vi "outline_boundaries_for_c_parameter.vi"(8 "Error In":errorcluster, 9 "Xi":T4, 10 "Sample":string, 11 "File Path":path) -> (0 "Error Out":errorcluster, 2 "Image":string, 3 "ROI":T1)   [LabVIEW 2019]
uses:
  xi_angles_enum_typedef.ctl
  image_property_cluster_typedef.ctl
  outline_boundaries_for_c_parameter_states_enum_typedef.ctl
  <vilib>/vision/NI_Vision_Development_Module.lvlib
panel:
  in  "Operator Value":sgl format="%.2f"
  in  "Operator":T2(ring)
  out "Image Properties":T3
  in  "Done":bool
  in  "Frame":i32(slide) min=0 max=19 step=1 scale=0.0..19.0
  out "Image":T5(plugin-control)
  # "Outline Boundaries for c-Parameter Determination"
  # "Use the open boundary selection tool to ouline grain boundaries that you wish to use for determining the c-parameter.\nRemember grains further from the center work the best for this task as they are more sensitive to the c-parameter."
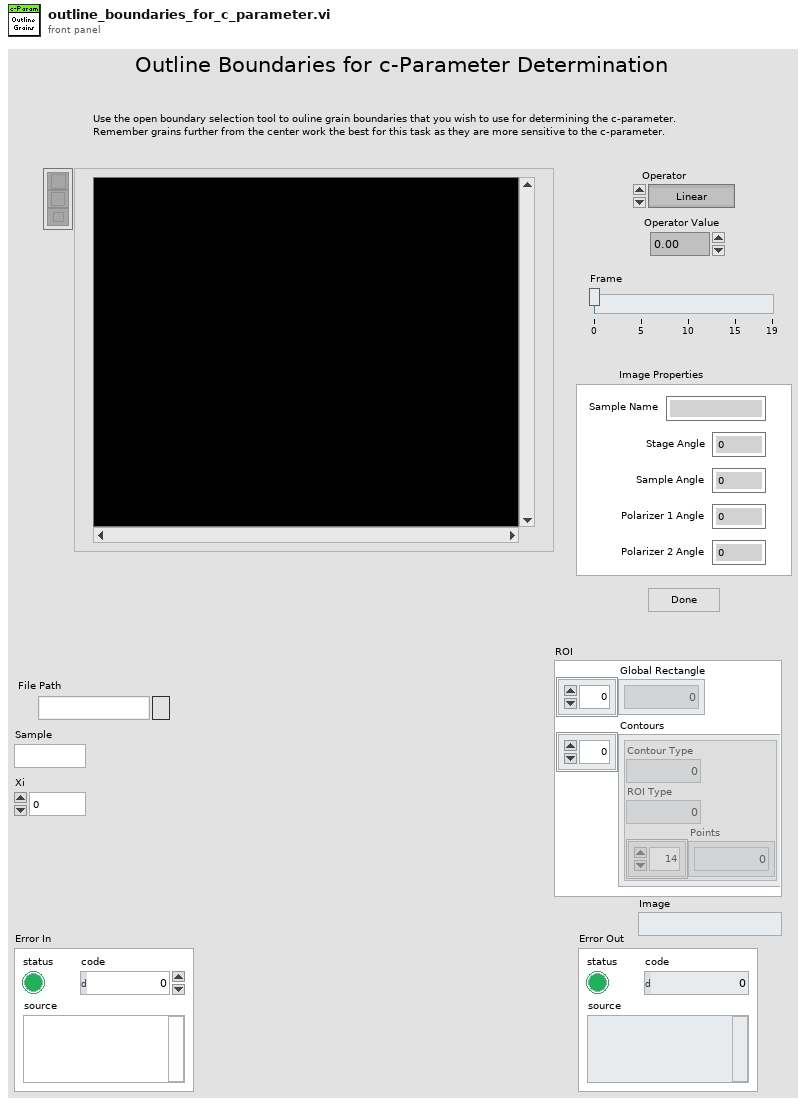
[diagram p1: front panel]
types:
  T1 = cluster{"Global Rectangle":i32[], "Contours":cluster{"Contour Type":u32, "ROI Type":u32, "Points":i32[]}[]}
  T2 = enum32{"Linear", "Log", "Exp", "Square", "Square root", "Power X", "Power 1/X"}
  T3 = typedef "image_property_cluster_typedef.ctl" = cluster{"Stage Angle":dbl, "Sample Angle":dbl, "Polarizer 1 Angle":dbl, "Polarizer 2 Angle":dbl, "Sample Name":string}
  T4 = typedef "xi_angles_enum_typedef.ctl" = enum16{"0", "45"}
  T5 = typedef "IMAQ Image.ctl" = refnum<image>
  T6 = typedef "outline_boundaries_for_c_parameter_states_enum_typedef.ctl" = enum16{"Enhance", "Plot Image", "Shutdown", "Wait", "Initialize", ""}
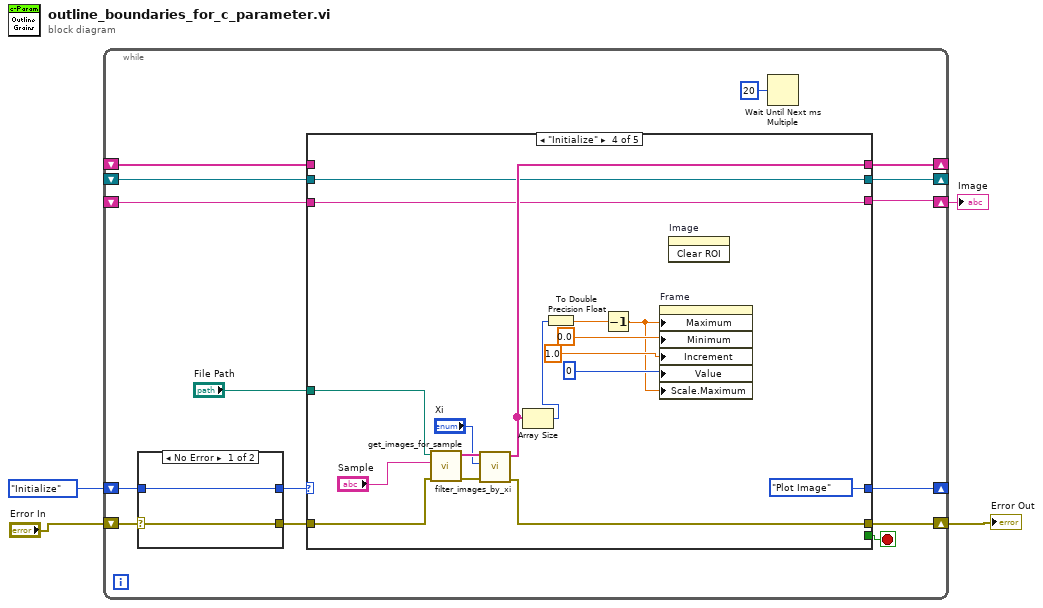
[diagram p0: block diagram]
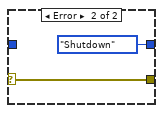
[diagram p2: hidden frame]
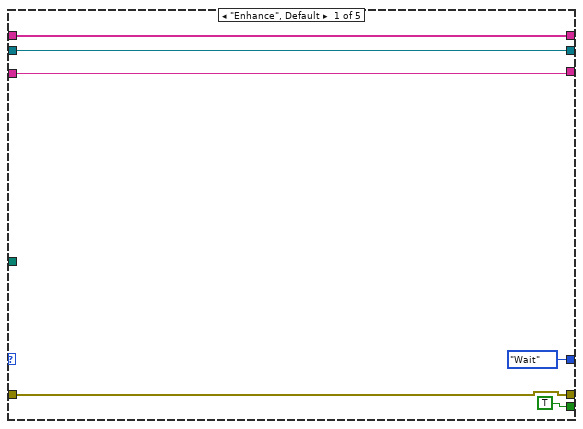
[diagram p3: hidden frame]
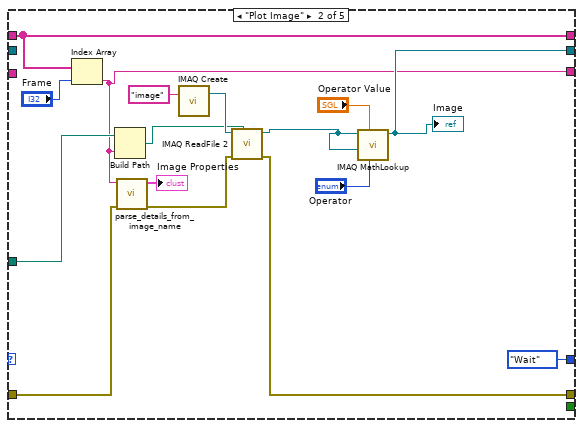
[diagram p4: hidden frame]
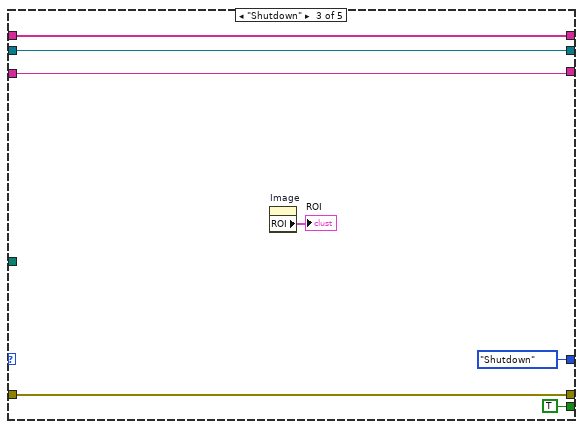
[diagram p5: hidden frame]
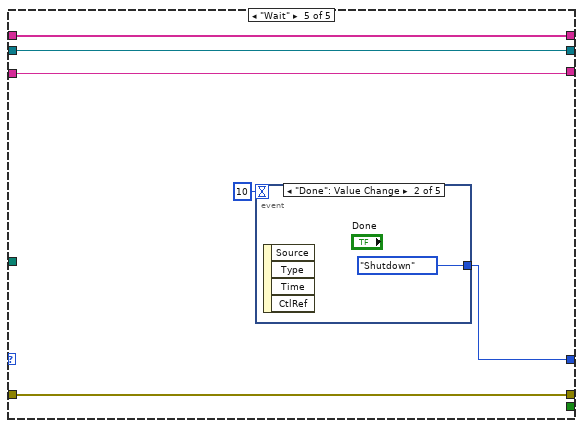
[diagram p6: hidden frame]
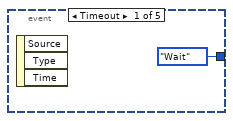
[diagram p7: hidden frame]
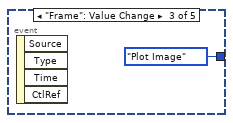
[diagram p8: hidden frame]
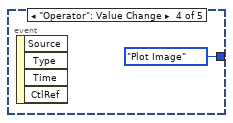
[diagram p9: hidden frame]
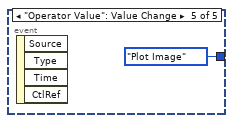
[diagram p10: hidden frame]
diagram:
  n1 = while {
    shift-right: [w16] -> _
    shift-left: outline_boundaries_for_c_parameter_states_enum_typedef."Initialize" -> [w19]
    shift-right: [w15] -> w2
    shift-left: "Error In" -> [w18]
    shift-right: [w13] -> _
    shift-left: _ -> [w12]
    shift-right: [w8] -> _
    shift-left: _ -> [w10]
    shift-right: [w6] -> w1
    shift-left: _ -> [w5]
    stop <- w14 stop-if-true
    n2 = case shown="No Error" w18 {
      selector: w18 -> [w20 w22]
      tunnel: [w21 outline_boundaries_for_c_parameter_states_enum_typedef."Shutdown"] -> w7
      tunnel: w19 -> [w21 _]
      tunnel: [w20 w22] -> w17
      frame No Error {
      }
      frame Error {
      }
    }
    n3 = case shown="\"Initialize\"" w7 {
      tunnel: w17 -> [w25 w35 w50 w65 w73]
      tunnel: [outline_boundaries_for_c_parameter_states_enum_typedef."Wait" outline_boundaries_for_c_parameter_states_enum_typedef."Wait" outline_boundaries_for_c_parameter_states_enum_typedef."Shutdown" outline_boundaries_for_c_parameter_states_enum_typedef."Plot Image" w74] -> w16
      tunnel: [w25 w40 w50 w59 w73] -> w15
      tunnel: [TRUE _ TRUE _ _] -> w14
      tunnel: [w27 w38 w52 w58 w72] -> w13
      tunnel: w12 -> [w27 w38 w52 _ w72]
      tunnel: "File Path" -> [_ w44 _ w57 _]
      tunnel: [w26 w31 w51 w56 w71] -> w8
      tunnel: w10 -> [w26 _ w51 w56 w71]
      tunnel: [w24 w30 w46 w53 w70] -> w6
      tunnel: w5 -> [w24 _ w46 w53 w70]
      frame "Enhance", Default {
      }
      frame "Plot Image" {
        n4 = Index Array(array=w38, index="Frame") -> (element=w30:string)
        n5 = Build Path(base path=w44, name or relative path=w30) -> (appended path=w41:path)
        n6 = call "parse_details_from_image_name.vi"("Error In"=w35, "Image Name"=w30) -> ("Error Out"=w36:errorcluster, "Image Properties"=→"Image Properties":T3)  [unwired: 8 in]
        n7 = call "IMAQ Create"("Image Name"="image") -> ("New Image"=w42:T5)  [unwired: 4 in, 1 out]
        n8 = call "IMAQ ReadFile 2"("File Path"=w41, "error in (no error)"=w36, "Image"=w42) -> ("error out"=w40:errorcluster, "Image Out"=w32:T5)  [unwired: 4 in, 3 out]
        n9 = call "IMAQ MathLookup"("Operator"="Operator", "X Value"="Operator Value", "Image Dst"=w32, "Image Src"=w32) -> ("Image Dst Out"=w31:T5)  [unwired: 6 in, 1 out]
        "Image" <- w31
      }
      frame "Shutdown" {
        n10 = property on="Image" class="ImageControl"() -> ("ROI"=→"ROI":T1)  [unwired: 2 in, 2 out]
      }
      frame "Initialize" {
        n11 = call "get_images_for_sample.vi"("Error In"=w65, "Sample"="Sample", "File Path"=w57) -> ("Error Out"=w68:errorcluster, "Image Names"=w67:string[])  [unwired: 7 in]
        n12 = call "filter_images_by_xi.vi"("Error In"=w68, "Xi"="Xi", "Image Names"=w67) -> ("Error Out"=w59:errorcluster, "Filtered Image Names"=w58:string[])  [unwired: 7 in]
        n13 = Array Size(array=w58) -> (size(s)=w61:i32)
        n14 = To Double Precision Float(number=w61) -> (double precision float=w55:dbl)
        n15 = Decrement(x=w55) -> (x-1=w54:dbl)
        n16 = property on="Frame" class="Slide (strict)"("Maximum"=w54, "Minimum"=0.0 ("Data Entry Limits:Minimum"), "Increment"=1.0 ("Data Entry Limits:Increment"), "Value"=0 ("Frame"), "Scale.Maximum"=w54) -> ()  [unwired: 2 in, 2 out]
        n17 = invoke on="Image" class="ImageControl" method="Clear ROI"() -> ()  [unwired: 3 in, 3 out]
      }
      frame "Wait" {
        n18 = event shown="[1] \"Done\": Value Change" {
          selector: _ -> [_ _ _ _ _]
          dyn-events: _ -> [_ _ _ _ _]
          timeout: 10 -> [_ _ _ _ _]
          tunnel: [outline_boundaries_for_c_parameter_states_enum_typedef."Wait" outline_boundaries_for_c_parameter_states_enum_typedef."Shutdown" outline_boundaries_for_c_parameter_states_enum_typedef."Plot Image" outline_boundaries_for_c_parameter_states_enum_typedef."Plot Image" outline_boundaries_for_c_parameter_states_enum_typedef."Plot Image"] -> w74
          event Timeout {
            n19 = event-data() -> ()  [unwired: 1 in, 3 out]
          }
          event "Done": Value Change {
            n20 = event-data() -> ()  [unwired: 1 in, 4 out]
          }
          event "Frame": Value Change {
            n21 = event-data() -> ()  [unwired: 1 in, 4 out]
          }
          event "Operator": Value Change {
            n22 = event-data() -> ()  [unwired: 1 in, 4 out]
          }
          event "Operator Value": Value Change {
            n23 = event-data() -> ()  [unwired: 1 in, 4 out]
          }
        }
      }
    }
    n24 = Wait Until Next ms Multiple(millisecond multiple=u32 20) -> ()  [unwired: 1 out]
  }
  "Error Out" <- w2
  "Image" <- w1
